vi "DLL Read Config.vi"(8 "error in (no error)":errorcluster, 11 "Phasor Data Concentrator in":refnum<class "Phasor Data Concentrator.lvclass">) -> (0 "error out":errorcluster, 3 "Phasor Data Concentrator out":refnum<class "Phasor Data Concentrator.lvclass">)   [LabVIEW 2013, in "PMU Recorder Light.lvlib" / "Phasor Data Concentrator.lvclass"]
doc: "Calls the DLL class to connect to the PDC."
uses:
  Phasor Data Concentrator.lvclass
  Statnett C37.118 DLL/Statnett C37.118 DLL.lvclass
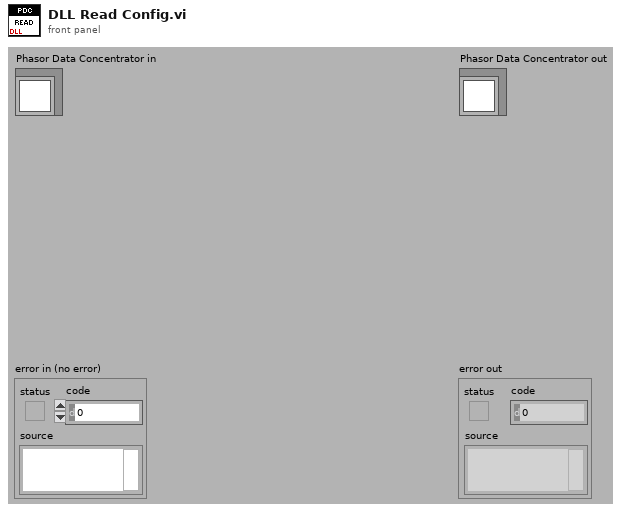
[diagram p1: front panel]
types:
  T1 = cluster{"Pseudo PDC ID":i32, "PMU Index":i32, "pmuconf out":cluster{"pmuid":i32, "nominalFrequency":sgl, "numberOfPhasors":i32, "numberOfAnalog":i32, "numberOfDigital":i32}, "Station Name":string, "Phasor Configuration":cluster{cluster{"type":u8, "format":u8, "dataIsScaled":u8, "@dummy control@":i8, "scalar":sgl}[], string[]}, "Analog Configuration":cluster{cluster{"Type":i32, "dataIsScaled":u8, "@dummy control@":i8, "@dummy control@":i8, "@dummy control@":i8, "userdefined_scalar":sgl}[], string[]}, "Digital Configuration":cluster{cluster{"normalBit":u8, "isValidBit":u8}[], string[]}}[]
  T2 = cluster{"LeapSecCorrection":i32, "LeapSecPending":u8, "ClockIsReliable":u8, "@dummy control@":i8, "@dummy control@":i8, "ClockErrorSec":sgl, "Year":i16, "Month":i16, "Day":i16, "Hour":i16, "Minute":i16, "Second":i16, "Ms":i16, "@dummy control@":i8, "@dummy control@":i8, "@dummy control@":i8, "@dummy control@":i8, "@dummy control@":i8, "@dummy control@":i8, "SecondOfCentury":dbl, "FramesPerSecond":sgl, "numberOfPMUs":i32}
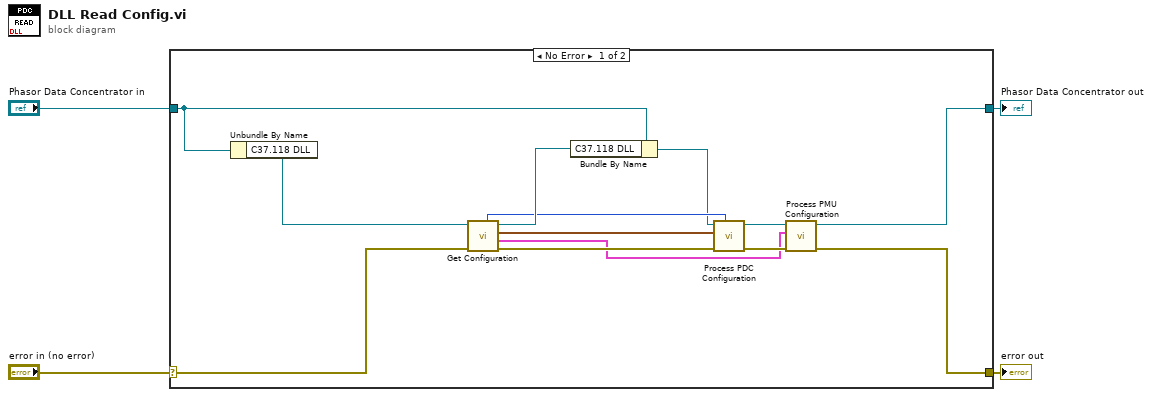
[diagram p0: block diagram]
diagram:
  n1 = case shown="No Error" "error in (no error)" {
    selector: "error in (no error)" -> [w12 w19]
    tunnel: [w14 w19] -> w3
    tunnel: [w15 w18] -> w1
    tunnel: "Phasor Data Concentrator in" -> [w17 w18]
    frame No Error {
      n2 = Unbundle By Name(w17) -> ("C37.118 DLL"=w13:refnum<class "Statnett C37.118 DLL.lvclass">)
      n3 = call "Get Configuration.vi"("error in (no error)"=w12, "Statnett C37.118 DLL in"=w13) -> ("error out"=w11:errorcluster, "PMU Configuration"=w5:T1, "PDC Configuration"=w10:T2, "Statnett C37.118 DLL out"=w16:refnum<class "Statnett C37.118 DLL.lvclass">, "Pseudo PDC ID"=w9:i32)  [unwired: 5 in]
      n4 = Bundle By Name(cluster=w17, "C37.118 DLL"=w16) -> (w8:refnum<class "Phasor Data Concentrator.lvclass">)
      n5 = call "Process PDC Configuration.vi"("Pseudo PDC ID"=w9, "error in (no error)"=w11, "PDC Configuration"=w10, "Phasor Data Concentrator in"=w8) -> ("error out"=w6:errorcluster, "Phasor Data Concentrator out"=w7:refnum<class "Phasor Data Concentrator.lvclass">)  [unwired: 6 in]
      n6 = call "Process PMU Configuration.vi"("error in (no error)"=w6, "PMU Configuration"=w5, "Phasor Data Concentrator in"=w7) -> ("error out"=w14:errorcluster, "Phasor Data Concentrator out"=w15:refnum<class "Phasor Data Concentrator.lvclass">)  [unwired: 7 in]
    }
    frame Error {
    }
  }
  "error out" <- w3
  "Phasor Data Concentrator out" <- w1
